vi "test14.2-MappingRelationshipByExternalRegistration_API_State.vi"() -> ()   [LabVIEW 2017, in "testcase-CSMBroadcast.lvclass"]
uses:
  testcase-CSMBroadcast.lvclass
  src/user.lib/_NEVSTOP/Communicable State Machine(CSM)/Communicable State Machine.lvlib
  <vilib>/addons/_JKI Toolkits/VI Tester/TestCase.llb/TestCase.lvclass
  C:/Program Files (x86)/National Instruments/LabVIEW 2017/vi.lib/addons/_JKI Toolkits/VI Tester/TestCase.llb/TestCase.lvclass
panel:
  out "Rules 1":T1(array[cluster])
  out "Status In Registry 1":string[](array[string])
  out "Rules 2":T1(array[cluster])
  out "Status In Registry 2":string[](array[string])
  out "Loop Count":i32
  out "Error Array":errorcluster[](array[cluster])
  out "TestCase out":refnum<class "testcase-CSMBroadcast.lvclass">
  in  "TestCase in":refnum<class "testcase-CSMBroadcast.lvclass">
  out "error out":errorcluster
  in  "error in (no error)":errorcluster
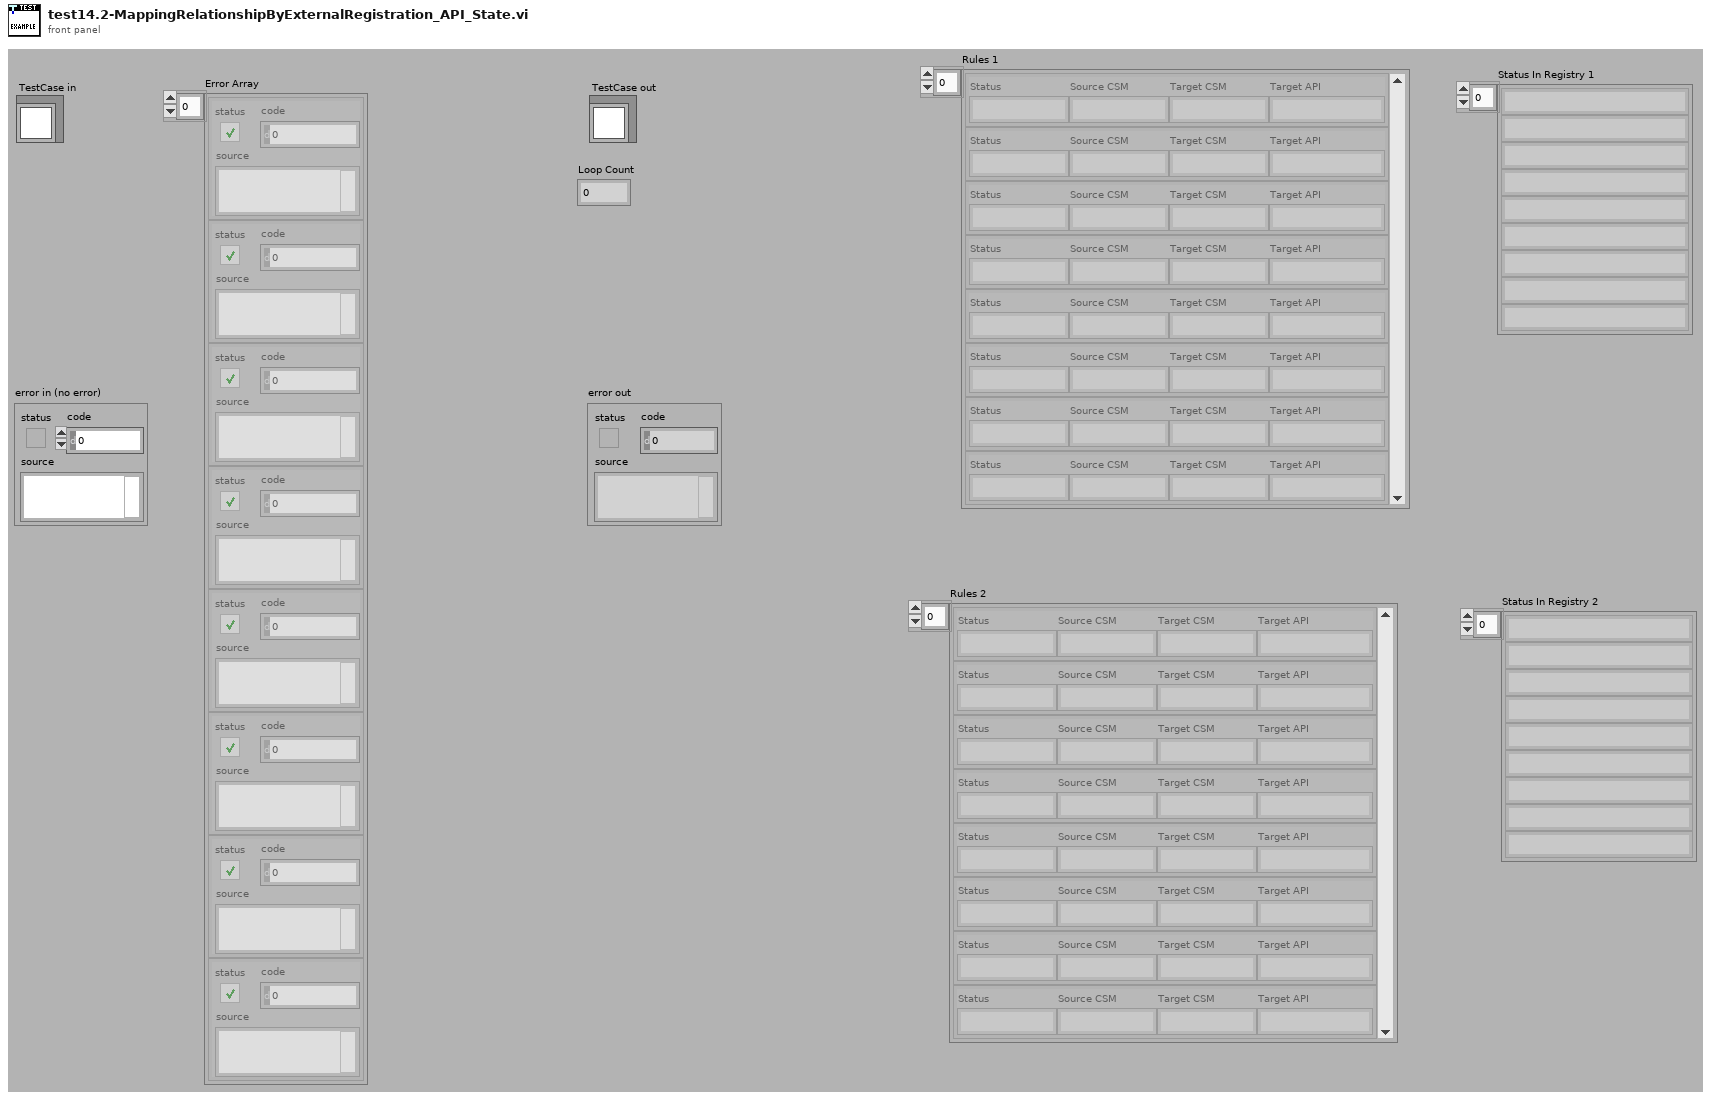
[diagram p1: front panel]
types:
  T1 = cluster{"Status":string, "Source CSM":string, "Target CSM":string, "Target API":string}[]
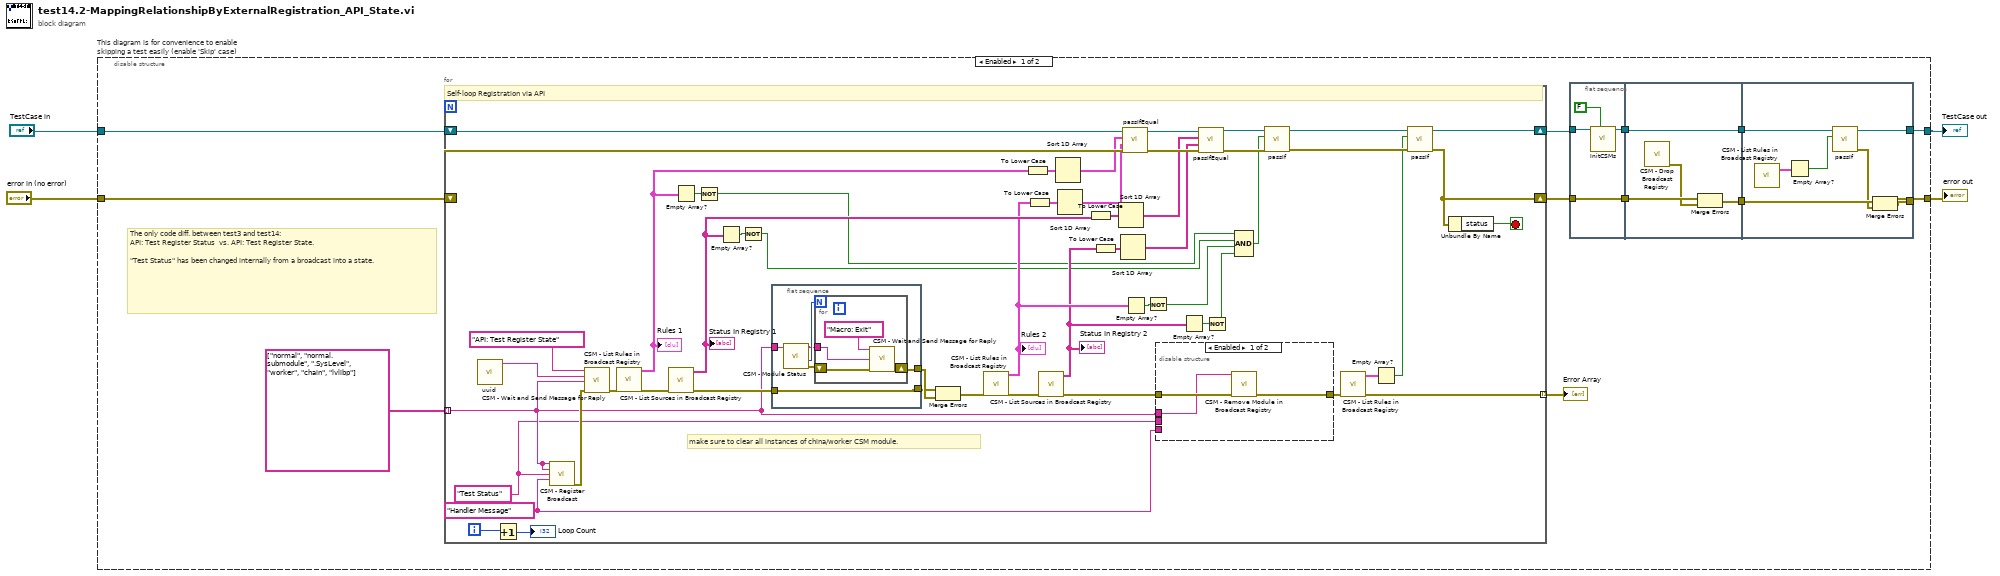
[diagram p0: block diagram]
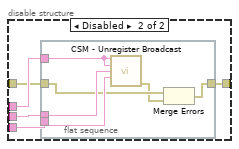
[diagram p2: hidden frame]
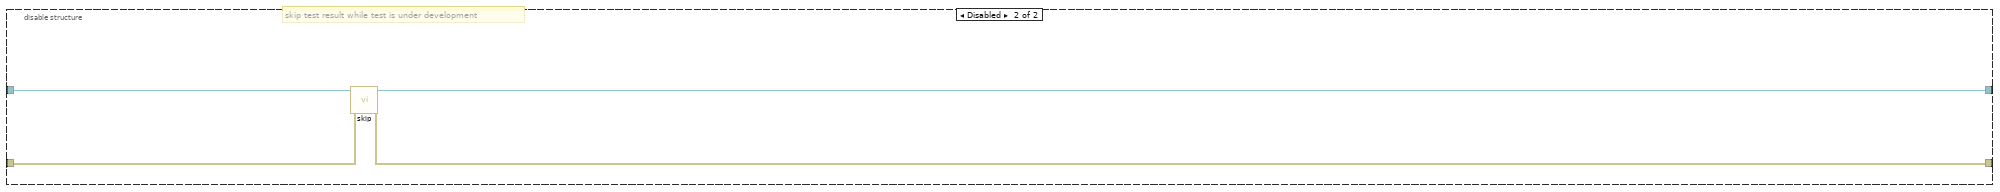
[diagram p3: hidden frame]
diagram:
  n1 = disable-structure "This diagram is for convenience to enable skipping a test easily (enable 'Skip' case)" shown="Enabled" {
    disable-tunnel: "TestCase in" -> [w16 w111]
    disable-tunnel: [w6 w109] -> w1
    disable-tunnel: [w5 w110] -> w3
    disable-tunnel: "error in (no error)" -> [w13 w108]
    frame Enabled {
      # "The only code diff. between test3 and test14:\nAPI: Test Register Status  vs. API: Test Register State.\n\n\"Test Status\" has been changed internally from a broadcast into a state."
      n2 = for {
        tunnel: string[] ["normal", "normal.submodule", ".SysLevel", "worker", "chain", "lvlibp"] -> [w42] mode=indexing
        shift-right: [w36] -> w10
        shift-left: w16 -> [w78]
        shift-right: [w34] -> w9
        shift-left: w13 -> [w77]
        tunnel: [w38] -> w15 mode=indexing
        i -> [w63]
        stop <- w76 stop-if-true
        w41 = "Handler Message" ("Response Message (If \"\", Same as Source Message)")
        w40 = "Test Status" ("Status")
        # "make sure to clear all instances of china/worker CSM module."
        # "Self-loop Registration via API"
        n3 = call "uuid.vi"() -> ("UUID"=w82:string)  [unwired: 11 in]
        n4 = Increment(x=w63) -> (x+1=→"Loop Count":i32)
        n5 = call "CSM - Register Broadcast.vi"("CSM Name(Empty for Broadcast Event)"=w42, "Source CSM Name (* as Default)"=w42, "Trigger"=w40, "API (If \"\", Same as Trigger)"=w41) -> ("error out"=w44:errorcluster)  [unwired: 10 in, 1 out]
        n6 = call "CSM - Wait and Send Message for Reply.vi"("State"="API: Test Register State", "Arguments (\"\")"=w82, "Target Module"=w42, "Error In (No Error)"=w44) -> ("error out"=w81:errorcluster)  [unwired: 8 in, 3 out]
        n7 = call "CSM - List Rules in Broadcast Registry.vi"("error in (no error)"=w81) -> ("error out"=w75:errorcluster, "Rule Entries"=w59:T1)  [unwired: 8 in, 1 out]
        "Rules 1" <- w59
        n8 = call "CSM - List Sources in Broadcast Registry.vi"("error in (no error)"=w75) -> ("error out"=w61:errorcluster, "Broadcast Names"=w56:string[])  [unwired: 9 in]
        "Status In Registry 1" <- w56
        n9 = Empty Array?(array=w59) -> (empty?=w58:bool)
        n10 = Not(x=w58) -> (.not. x?=w51:bool)
        n11 = Empty Array?(array=w56) -> (empty?=w57:bool)
        n12 = Not(x=w57) -> (.not. x?=w50:bool)
        n13 = flat-sequence {
          tunnel: [w103] -> w80
          tunnel: w42 -> [w101]
          tunnel: [w100] -> w60
          tunnel: w61 -> [w100]
          frame #0 {
            n14 = call "CSM - Module Status.vi"("CSM Name"=w101) -> ("error out"=w98:errorcluster, "#Nodes"=w102:i32, "CSM Name (Dup)"=w99:string)  [unwired: 6 in, 2 out]
            n15 = for {
              N: w102 -> [_]
              tunnel: w99 -> [w105]
              shift-right: [w106] -> w103
              shift-left: w98 -> [w104]
              n16 = call "CSM - Wait and Send Message for Reply.vi"("State"="Macro: Exit", "Target Module"=w105, "Error In (No Error)"=w104) -> ("error out"=w106:errorcluster)  [unwired: 9 in, 3 out]
            }
          }
        }
        n17 = Merge Errors(w60, w80) -> (w79:errorcluster)
        n18 = call "CSM - List Rules in Broadcast Registry.vi"("error in (no error)"=w79) -> ("error out"=w74:errorcluster, "Rule Entries"=w54:T1)  [unwired: 8 in, 1 out]
        "Rules 2" <- w54
        n19 = To Lower Case(string=w59) -> (all lower case string=w73:T1)
        n20 = To Lower Case(string=w54) -> (all lower case string=w72:T1)
        n21 = call "CSM - List Sources in Broadcast Registry.vi"("error in (no error)"=w74) -> ("error out"=w43:errorcluster, "Broadcast Names"=w52:string[])  [unwired: 9 in]
        "Status In Registry 2" <- w52
        n22 = Sort 1D Array(array=w73) -> (sorted array=w71:T1)
        n23 = Sort 1D Array(array=w72) -> (sorted array=w70:T1)
        n24 = To Lower Case(string=w56) -> (all lower case string=w67:string[])
        n25 = To Lower Case(string=w52) -> (all lower case string=w66:string[])
        n26 = Sort 1D Array(array=w67) -> (sorted array=w65:string[])
        n27 = Sort 1D Array(array=w66) -> (sorted array=w64:string[])
        n28 = call-dynamic "passIfEqual.vi"("error in (no error)"=w77, "y"=w70, "x"=w71, "TestCase in"=w78) -> ("error out"=w68:errorcluster, "TestCase out"=w69:refnum<class "testcase-CSMBroadcast.lvclass">)  [unwired: 6 in]
        n29 = Empty Array?(array=w54) -> (empty?=w55:bool)
        n30 = Not(x=w55) -> (.not. x?=w49:bool)
        n31 = disable-structure shown="Enabled" {
          disable-tunnel: w43 -> [w86 w88]
          disable-tunnel: [w85 w87] -> w39
          disable-tunnel: w42 -> [w84 w89]
          disable-tunnel: w40 -> [_ w91]
          disable-tunnel: w41 -> [_ w90]
          frame Enabled {
            n32 = call "CSM - Remove Module in Broadcast Registry.vi"("CSM Name"=w84, "Error In"=w86) -> ("error out"=w85:errorcluster)  [unwired: 12 in, 1 out]
          }
          frame Disabled {
            n33 = flat-sequence {
              tunnel: w91 -> [w97]
              tunnel: w90 -> [w96]
              tunnel: w89 -> [w95]
              tunnel: w88 -> [w94]
              tunnel: [w92] -> w87
              frame #0 {
                n34 = call "CSM - Unregister Broadcast.vi"("CSM Name(Empty for Broadcast Event)"=w95, "Source CSM Name (* as Default)"=w95, "Trigger"=w97, "API (\"*\" as Default)"=w96) -> ("error out"=w93:errorcluster)  [unwired: 10 in, 1 out]
                n35 = Merge Errors(w94, w93) -> (w92:errorcluster)
              }
            }
          }
        }
        n36 = Empty Array?(array=w52) -> (empty?=w53:bool)
        n37 = call-dynamic "passIfEqual.vi"("error in (no error)"=w68, "y"=w64, "x"=w65, "TestCase in"=w69) -> ("error out"=w46:errorcluster, "TestCase out"=w47:refnum<class "testcase-CSMBroadcast.lvclass">)  [unwired: 6 in]
        n38 = Not(x=w53) -> (.not. x?=w48:bool)
        n39 = Compound Arithmetic op=AND(w51, w50, w49, w48) -> (w45:bool)
        n40 = call-dynamic "passIf.vi"("error in (no error)"=w46, "pass"=w45, "TestCase in"=w47) -> ("error out"=w35:errorcluster, "TestCase out"=w37:refnum<class "testcase-CSMBroadcast.lvclass">)  [unwired: 7 in]
        n41 = call "CSM - List Rules in Broadcast Registry.vi"("error in (no error)"=w39) -> ("error out"=w38:errorcluster, "Rule Entries"=w33:T1)  [unwired: 8 in, 1 out]
        n42 = Empty Array?(array=w33) -> (empty?=w32:bool)
        n43 = call-dynamic "passIf.vi"("error in (no error)"=w35, "pass"=w32, "TestCase in"=w37) -> ("error out"=w34:errorcluster, "TestCase out"=w36:refnum<class "testcase-CSMBroadcast.lvclass">)  [unwired: 7 in]
        n44 = Unbundle By Name(w34) -> ("status"=w76:bool)
      }
      "Error Array" <- w15
      n45 = flat-sequence {
        tunnel: w10 -> [w20]
        tunnel: [w19] -> w12
        tunnel: [w18] -> w11
        tunnel: w9 -> [w18]
        tunnel: w12 -> [w24]
        tunnel: w11 -> [w23]
        tunnel: [w24] -> w8
        tunnel: [w22] -> w7
        tunnel: [w26] -> w5
        tunnel: [w28] -> w6
        tunnel: w8 -> [w29]
        tunnel: w7 -> [w31]
        frame #0 {
          n46 = call "InitCSMs.vi"("Enable building lvlibp?"=FALSE, "testcase-CSMStatus in"=w20) -> ("testcase-CSMStatus out"=w19:refnum<class "testcase-CSMBroadcast.lvclass">)  [unwired: 8 in, 1 out]
        }
        frame #1 {
          n47 = call "CSM - Drop Broadcast Registry.vi"() -> ("error out"=w21:errorcluster)  [unwired: 15 in]
          n48 = Merge Errors(w23, w21) -> (w22:errorcluster)
        }
        frame #2 {
          n49 = call "CSM - List Rules in Broadcast Registry.vi"() -> ("Rule Entries"=w30:T1)  [unwired: 9 in, 2 out]
          n50 = Empty Array?(array=w30) -> (empty?=w27:bool)
          n51 = call-dynamic "passIf.vi"("pass"=w27, "TestCase in"=w29) -> ("error out"=w25:errorcluster, "TestCase out"=w28:refnum<class "testcase-CSMBroadcast.lvclass">)  [unwired: 8 in]
          n52 = Merge Errors(w31, w25) -> (w26:errorcluster)
        }
      }
    }
    frame Disabled {
      # "skip test result while test is under development"
      n53 = call <vilib>:"skip.vi"("error in (no error)"=w108, "TestCase in"=w111) -> ("error out"=w110:errorcluster, "TestCase out"=w109:refnum<class "testcase-CSMBroadcast.lvclass">)  [unwired: 8 in]
    }
  }
  "error out" <- w3
  "TestCase out" <- w1
